vi "1L09-num1D_format-vers-txt_1D.vi"(8 "type":T1, 9 "1D( num)":dbl[](array[numeric])) -> (3 "1D (ch)":string[](array[string]))   [LabVIEW 2010, in "lv_01.lvlib"]
uses:
  lv_01.lvlib
  type format.ctl
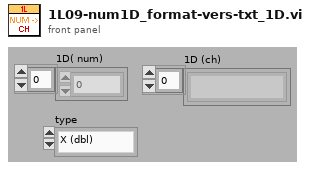
[diagram p1: front panel]
types:
  T1 = typedef "lv_01.lvlib/type format.ctl" = enum16{"X (dbl)", "P (Proba)", "N (entier)", "S (Scient.)"}
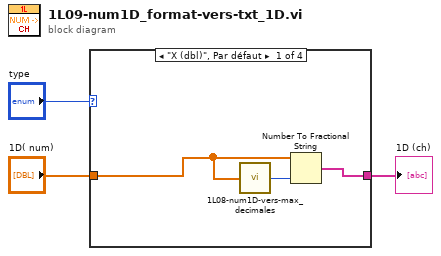
[diagram p0: block diagram]
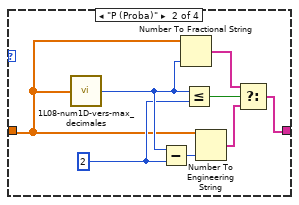
[diagram p2: hidden frame]
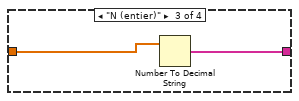
[diagram p3: hidden frame]
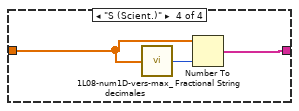
[diagram p4: hidden frame]
diagram:
  n1 = case shown="\"X (dbl)\", Par défaut" "type" {
    tunnel: "1D( num)" -> [w5 w7 w16 w17]
    tunnel: [w4 w8 w15 w18] -> w2
    frame "X (dbl)", Default {
      n2 = call "1L08-num1D-vers-max_decimales.vi"("num. déc. (1D)"=w5) -> ("Max déc."=w6:i32)
      n3 = Number To Fractional String(number=w5, precision (6)=w6) -> (F-format string=w4:string[])  [unwired: 2 in]
    }
    frame "P (Proba)" {
      w10 = 2 ("y")
      n4 = call "1L08-num1D-vers-max_decimales.vi"("num. déc. (1D)"=w7) -> ("Max déc."=w11:i32)
      n5 = Subtract(x=w11, y=w10) -> (x-y=w9:i32)
      n6 = Number To Fractional String(number=w7, precision (6)=w11) -> (F-format string=w13:string[])  [unwired: 2 in]
      n7 = Less Or Equal?(x=w11, y=w10) -> (x <= y?=w12:bool)
      n8 = Number To Engineering String(2:w9, 4:w7) -> (0:w14:string[])  [unwired: 2 in]
      n9 = Select(t=w13, s=w12, f=w14) -> (s? t:f=w8:string[])
    }
    frame "N (entier)" {
      n10 = Number To Decimal String(number=w16) -> (decimal integer string=w15:string[])  [unwired: 1 in]
    }
    frame "S (Scient.)" {
      n11 = call "1L08-num1D-vers-max_decimales.vi"("num. déc. (1D)"=w17) -> ("Max déc."=w19:i32)
      n12 = Number To Fractional String(number=w17, precision (6)=w19) -> (F-format string=w18:string[])  [unwired: 2 in]
    }
  }
  "1D (ch)" <- w2
